vi "Database.Handler-NewData.vi"(8 "error in":errorcluster, 10 "Data":T1={"Status"=0, "Ref1"="9998887770", "Serial1"="12345679", "Ref2"="", "Serial2"="", "Values"=[1.0, 2.0, 1.0, 1.0, 1.0, 4.0, 5.0, 1.0]} {"Values" format="%.3f"}, 11 "Idx":i32) -> (0 "error out":errorcluster, 2 "Saved":bool)   [LabVIEW 2016]
doc: "Go to DB->WriteStationValues action\nReturn boolean flag to show if data was saved to DB successfully\n\nWabco 2017 All right reserved\nAuthor: maciej.szupienko@wabco-auto.com"
uses:
  Drivers/PLC/LowLevel/PLC.DataBlock.PLCvalues.ctl
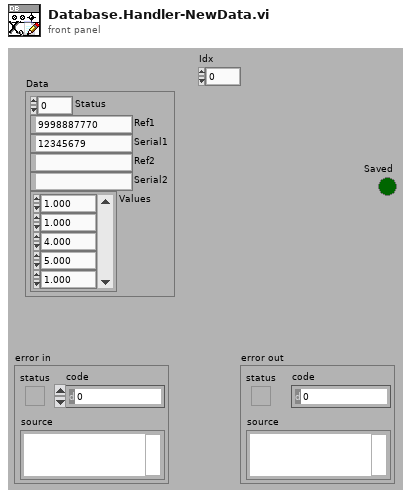
[diagram p1: front panel]
types:
  T1 = typedef "PLC.DataBlock.PLCvalues.ctl" = cluster{"Status":u8, "Ref1":string, "Serial1":string, "Ref2":string, "Serial2":string, "Values":sgl[]}
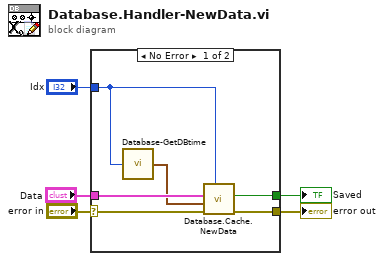
[diagram p0: block diagram]
diagram:
  n1 = case shown="No Error" "error in" {
    selector: "error in" -> [w11 w12]
    tunnel: [w10 w12] -> w4
    tunnel: "Data" -> [w9 _]
    tunnel: "Idx" -> [w7 _]
    tunnel: [w6 _] -> w1
    frame No Error {
      n2 = call "Database-GetDBtime.vi"("Idx"=w7) -> ("DbTime"=w8:timestamp)
      n3 = call "Database.Cache.NewData.vi"("Idx"=w7, "error in"=w11, "DBtime"=w8, "Data"=w9) -> ("error out"=w10:errorcluster, "Data saved"=w6:bool)  [unwired: 6 in]
    }
    frame Error {
    }
  }
  "error out" <- w4
  "Saved" <- w1
